vi "4p2_HW_Task2_UCweesesr.vi"() -> ()   [LabVIEW 2016]
panel:
  out "T (in C)":dbl
  in  "Beta":dbl
  in  "R_o":dbl
  in  "R":dbl
  in  "T_o":dbl
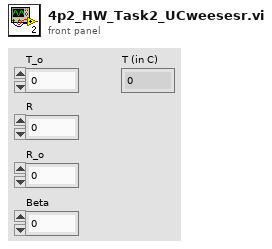
[diagram p1: front panel]
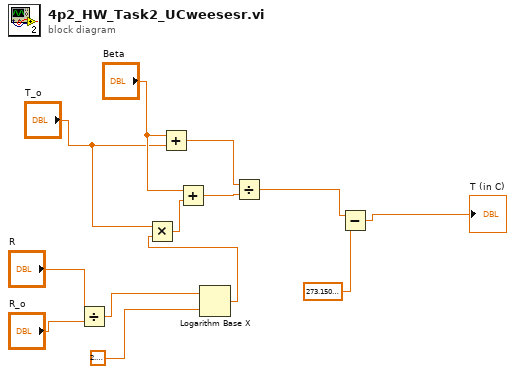
[diagram p0: block diagram]
diagram:
  n1 = Divide(x="R", y="R_o") -> (x/y=w2:dbl)
  n2 = Add(x="Beta", y="T_o") -> (x+y=w13:dbl)
  n3 = Logarithm Base X(1:2.718281828459045, 2:w2) -> (0:w1:dbl)
  n4 = Multiply(x="T_o", y=w1) -> (x*y=w4:dbl)
  n5 = Add(x="Beta", y=w4) -> (x+y=w9:dbl)
  n6 = Divide(x=w13, y=w9) -> (x/y=w12:dbl)
  n7 = Subtract(x=w12, y=273.1500000000001) -> (x-y=→"T (in C)":dbl)
